vi "Log.vi"   [LabVIEW 2021, in "BT.lvlib"]
uses:
  BT.lvlib
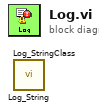
[diagram p0: block diagram]
diagram:
  n1 = call "Log_String.vi"() -> ()  [unwired: 11 in, 1 out]
  n2 = call "Log_StringClass.vi"() -> ()  [unwired: 11 in, 1 out]
